vi "CAN Wrapper.vi"(5 "Signal Write":dbl, 7 "States":T1=enum."Close", 8 "error in":errorcluster, 9 "Setting":T2={"Termination"=1, "Baud Rate"=125000, "Interface"="CAN1", "XNET Database"="can_messages_818", "ECU"="GIP\ncan_messages_818"} {"Termination" items=["Off", "On"]}, 10 "Tx Signal In":string="GIP_TestMode.GIP_TestModeFlag", 11 "Rx Signal In":string) -> (0 "error out":errorcluster, 3 "Signal out":dbl=nan)   [LabVIEW 2021, in "CAN wrapper.lvlib"]
uses:
  CAN wrapper.lvlib
  Private Controls/Setting.ctl
  Private Controls/CAN States.ctl
  Private Controls/Local Variables.ctl
  <vilib>/JDP Science/JSONtext/Next JSON Value.vi
  <vilib>/JDP Science/JSONtext/String Subset.vi
  <vilib>/JDP Science/JSONtext/Parsing/Advance past next JSON Value (inlined COPY).vi
  <vilib>/JDP Science/JSONtext/Parsing/Advance past whitespace.vi
  <vilib>/JDP Science/JSONtext/Parsing/Advance past String.vi
  <vilib>/JDP Science/JSONtext/Parsing/Advance past Number.vi
  <vilib>/JDP Science/JSONtext/Parsing/Advance past Line Ending.vi
  <vilib>/xnet/xnet.llb/XNET Create Session (Signal Input Single-point).vi
  <vilib>/xnet/xnet.llb/XNET Read (Signal Single-point).vi
  <vilib>/xnet/xnet.llb/XNET Create Session (Signal Output Single-point).vi
  <vilib>/JDP Science/JSONtext/Parsing/Parse Full Path or Item Name.vi
  <vilib>/JDP Science/JSONtext/Parsing/Advance past Array.vi
  <vilib>/JDP Science/JSONtext/Parsing/Advance past Object.vi
  <vilib>/JDP Science/JSONtext/support/Error Cluster From Code.vi
  <vilib>/JDP Science/JSONtext/Offset/Find Item Locations by Path.vi
  <vilib>/xnet/xnet.llb/XNET Write (Signal Single-point).vi
  <resource>/objmgr/xnet.rc
  <vilib>/JDP Science/JSONtext/JSONtext.lvlib
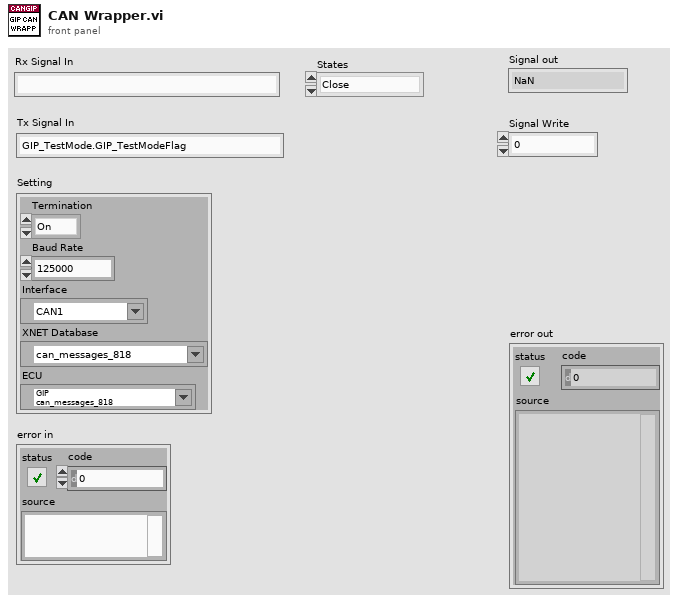
[diagram p1: front panel]
types:
  T1 = typedef "CAN wrapper.lvlib/CAN States.ctl" = enum16{"Init", "Rx Sess", "Tx Sess", "Read Signals", "Write Signals", "Close"}
  T2 = typedef "CAN wrapper.lvlib/Setting.ctl" = cluster{"Termination":u32, "Baud Rate":u64, "Interface":refnum<k21>, "XNET Database":refnum<k21>, "ECU":refnum<k21>}
  T3 = typedef "CAN wrapper.lvlib/Local Variables.ctl" = cluster{"Rx session":refnum<k21>, "Tx session":refnum<k21>, "Tx Data":dbl[], "JSON":string, "Tx Sigs":refnum<k21>[], "Rx Sigs":refnum<k21>[]}
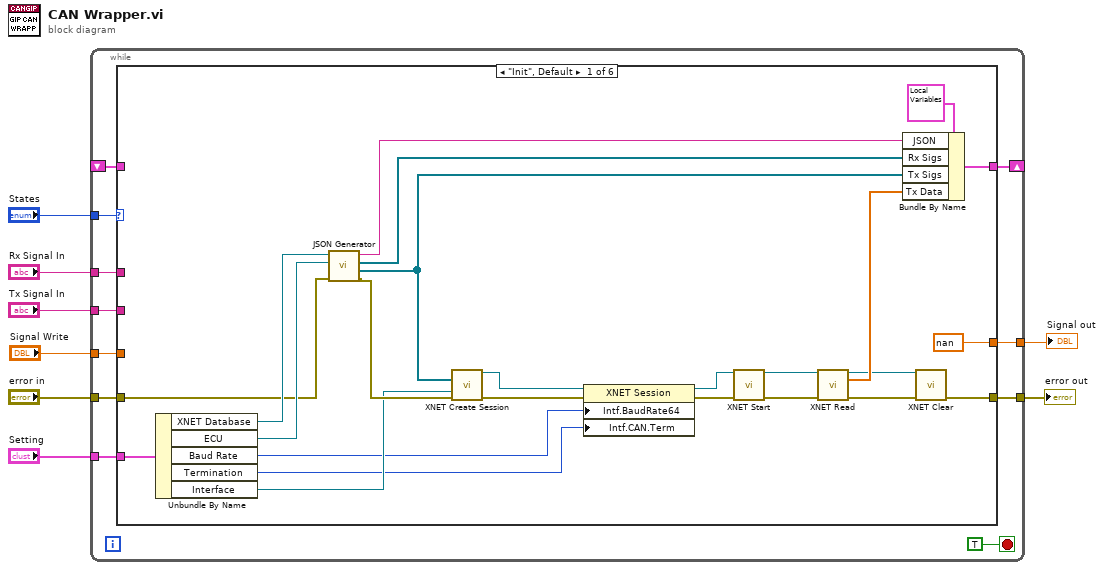
[diagram p0: block diagram]
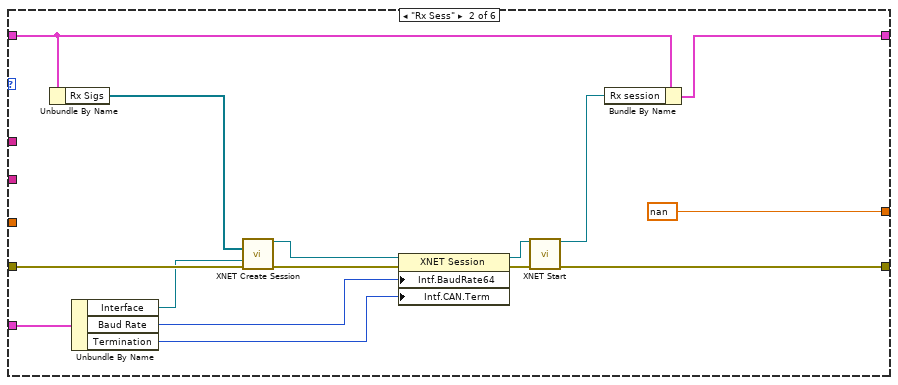
[diagram p2: hidden frame]
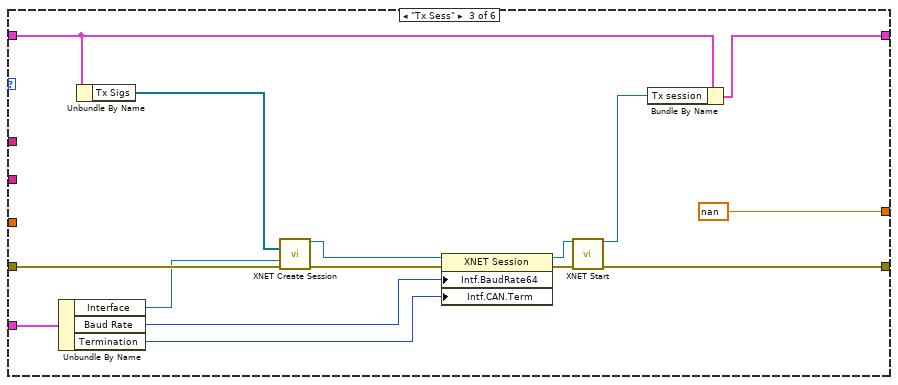
[diagram p3: hidden frame]
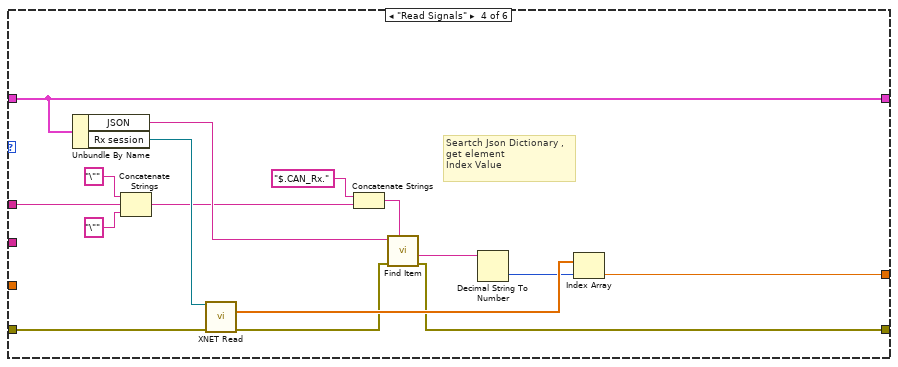
[diagram p4: hidden frame]
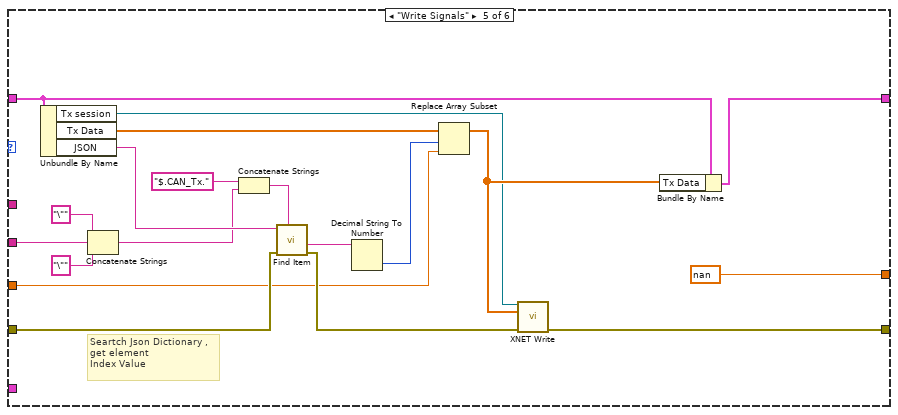
[diagram p5: hidden frame]
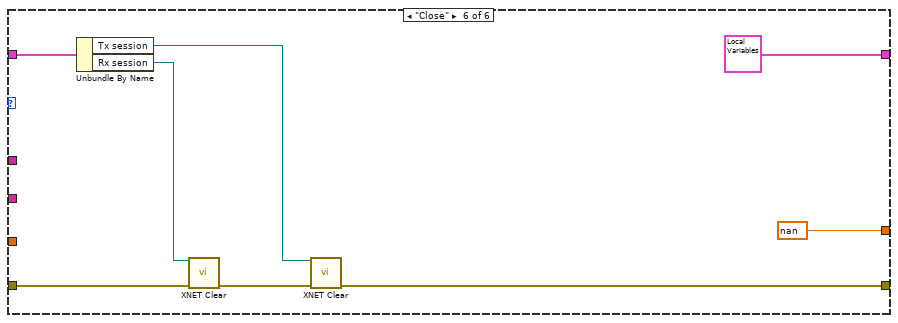
[diagram p6: hidden frame]
diagram:
  n1 = while {
    tunnel: "States" -> [w18]
    tunnel: "error in" -> [w17]
    tunnel: [w16] -> w7
    shift-right: [w15] -> _
    shift-left: _ -> [w14]
    tunnel: "Setting" -> [w13]
    tunnel: "Rx Signal In" -> [w12]
    tunnel: [w11] -> w3
    tunnel: "Signal Write" -> [w10]
    tunnel: "Tx Signal In" -> [w9]
    stop <- TRUE stop-if-true
    n2 = case shown="\"Init\", Default" w18 {
      tunnel: w17 -> [w31 w50 w68 w89 w102 w116]
      tunnel: [w21 w48 w64 w80 w90 w113] -> w16
      tunnel: [w30 w58 w65 w87 w96 T3 {"Rx session"="", "Tx session"="", "Tx Data"=[], "JSON"="{\n  \"CAN_Rx\":{\n    \"GIP_GetPartNumber.lChar0\":0,\n    \"GIP_GetPartNumber.lChar1\":1,\n    \"GIP_GetPartNumber.lChar2\":2,\n    \"GIP_GetPartNumber.lChar3\":3,\n    \"GIP_GetPartNumber.lChar4\":4,\n    \"GIP_GetPartNumber.lChar5\":5,\n    \"GIP_GetPartNumber.lChar6\":6,\n    \"GIP_GetPartNumber.lChar7\":7,\n    \"GIP_GetPartNumber.rChar0\":8,\n    \"GIP_GetPartNumber.rChar1\":9,\n    \"GIP_GetSerialNumber.vendorChar0\":10,\n    \"GIP_GetSerialNumber.vendorChar1\":11,\n    \"GIP_GetSerialNumber.vendorChar2\":12,\n    \"GIP_GetSerialNumber.weekAndSerial\":13,\n    \"GIP_Grid_ActiveEnergyExported.GIP_Grid_ActiveEnergyExported_L1\":14,\n    \"GIP_Grid_ActiveEnergyExported.GIP_Grid_ActiveEnergyExported_L2\":15,\n    \"GIP_Grid_ActiveEnergyImported.GIP_Grid_ActiveEnergyImported_L1\":16,\n    \"GIP_Grid_ActiveEnergyImported.GIP_Grid_ActiveEnergyImported_L2\":17,\n    \"GIP_Grid_Power.GIP_Grid_ActivePower_L1\":18,\n    \"GIP_Grid_Power.GIP_Grid_ActivePower_L2\":19,\n    \"GIP_Grid_Power.GIP_Grid_ReactivePower_L1\":20,\n    \"GIP_Grid_Power.GIP_Grid_ReactivePower_L2\":21,\n    \"GIP_Grid_TotalActiveEnergy.GIP_Grid_TotalActiveEnergyExported\":22,\n    \"GIP_Grid_TotalActiveEnergy.GIP_Grid_TotalActiveEnergyImported\":23,\n    \"GIP_Load_ActiveEnergyExported.GIP_Load_ActiveEnergyExported_L1\":24,\n    \"GIP_Load_ActiveEnergyExported.GIP_Load_ActiveEnergyExported_L2\":25,\n    \"GIP_Load_ActiveEnergyImported.GIP_Load_ActiveEnergyImported_L1\":26,\n    \"GIP_Load_ActiveEnergyImported.GIP_Load_ActiveEnergyImported_L2\":27,\n    \"GIP_Load_Power.GIP_Load_ActivePower_L1\":28,\n    \"GIP_Load_Power.GIP_Load_ActivePower_L2\":29,\n    \"GIP_Load_Power.GIP_Load_ReactivePower_L1\":30,\n    \"GIP_Load_Power.GIP_Load_ReactivePower_L2\":31,\n    \"GIP_Load_TotalActiveEnergy.GIP_Load_TotalActiveEnergyExported\":32,\n    \"GIP_Load_TotalActiveEnergy.GIP_Load_TotalActiveEnergyImported\":33,\n    \"GIP_Status.GIP_Relay_State\":34,\n    \"GIP_Status.GIP_State\":35\n  },\n  \"CAN_Tx\":{\n    \"GIP_ManufacturingControl.ESP32Comms\":0,\n    \"GIP_ManufacturingControl.FaultLED\":1,\n    \"GIP_ManufacturingControl.Relay\":2,\n    \"GIP_ManufacturingControl.ST8500Comms\":3,\n    \"GIP_ManufacturingControl.StatusLED\":4,\n    \"GIP_SetPartNumber.lChar0\":5,\n    \"GIP_SetPartNumber.lChar1\":6,\n    \"GIP_SetPartNumber.lChar2\":7,\n    \"GIP_SetPartNumber.lChar3\":8,\n    \"GIP_SetPartNumber.lChar4\":9,\n    \"GIP_SetPartNumber.lChar5\":10,\n    \"GIP_SetPartNumber.lChar6\":11,\n    \"GIP_SetPartNumber.lChar7\":12,\n    \"GIP_SetPartNumber.rChar0\":13,\n    \"GIP_SetPartNumber.rChar1\":14,\n    \"GIP_SetSerialNumber.vendorChar0\":15,\n    \"GIP_SetSerialNumber.vendorChar1\":16,\n    \"GIP_SetSerialNumber.vendorChar2\":17,\n    \"GIP_SetSerialNumber.weekAndSerial\":18,\n    \"GIP_SetTestedFlag.GIP_TestedFlag\":19,\n    \"GIP_TestMode.GIP_TestModeFlag\":20\n  }\n}", "Tx Sigs"=[], "Rx Sigs"=[]}] -> w15
      tunnel: w14 -> [_ w49 w67 w87 w99 w115]
      tunnel: w13 -> [w32 w47 w62 _ _ _]
      tunnel: w12 -> [_ _ _ w75 _ _]
      tunnel: [nan nan nan w85 nan nan] -> w11
      tunnel: w10 -> [_ _ _ _ w100 _]
      tunnel: w9 -> [_ _ _ _ w94 _]
      frame "Init", Default {
        n3 = Unbundle By Name(w32) -> ("XNET Database"=w42:refnum<k21>, "ECU"=w41:refnum<k21>, "Baud Rate"=w34:u64, "Termination"=w33:u32, "Interface"=w39:refnum<k21>)
        n4 = call "JSON Generator.vi"("error in (no error)"=w31, "ECU"=w41, "XNET Database"=w42) -> ("error out"=w40:errorcluster, "Tx Sigs"=w23:refnum<k21>[], "Rx Sigs"=w24:refnum<k21>[], "JSON"=w26:string)  [unwired: 5 in]
        n5 = call-poly <vilib>:"XNET Create Session.vi"("signal list"=w23, "interface"=w39, "error in (no error)"=w40) -> ("session out"=w37:refnum<k21>, "error out"=w35:errorcluster)  [unwired: 11 out]
        n6 = property class="XNET Session"(reference=w37, error in=w35, "Intf.BaudRate64"=w34, "Intf.CAN.Term"=w33) -> (reference out=w36:refnum<k21>, error out=w38:errorcluster)
        n7 = call <vilib>:"XNET Start.vi"("session in"=w36, "error in (no error)"=w38) -> ("session out"=w28:refnum<k21>, "error out"=w29:errorcluster)  [unwired: 12 in]
        n8 = call-poly <vilib>:"XNET Read.vi"("session in"=w28, "error in (no error)"=w29) -> ("session out"=w20:refnum<k21>, "data"=w27:dbl[], "error out"=w22:errorcluster)  [unwired: 11 out]
        n9 = Bundle By Name(cluster=T3 {"Rx session"="", "Tx session"="", "Tx Data"=[], "JSON"="{\n  \"CAN_Rx\":{\n    \"GIP_GetPartNumber.lChar0\":0,\n    \"GIP_GetPartNumber.lChar1\":1,\n    \"GIP_GetPartNumber.lChar2\":2,\n    \"GIP_GetPartNumber.lChar3\":3,\n    \"GIP_GetPartNumber.lChar4\":4,\n    \"GIP_GetPartNumber.lChar5\":5,\n    \"GIP_GetPartNumber.lChar6\":6,\n    \"GIP_GetPartNumber.lChar7\":7,\n    \"GIP_GetPartNumber.rChar0\":8,\n    \"GIP_GetPartNumber.rChar1\":9,\n    \"GIP_GetSerialNumber.vendorChar0\":10,\n    \"GIP_GetSerialNumber.vendorChar1\":11,\n    \"GIP_GetSerialNumber.vendorChar2\":12,\n    \"GIP_GetSerialNumber.weekAndSerial\":13,\n    \"GIP_Grid_ActiveEnergyExported.GIP_Grid_ActiveEnergyExported_L1\":14,\n    \"GIP_Grid_ActiveEnergyExported.GIP_Grid_ActiveEnergyExported_L2\":15,\n    \"GIP_Grid_ActiveEnergyImported.GIP_Grid_ActiveEnergyImported_L1\":16,\n    \"GIP_Grid_ActiveEnergyImported.GIP_Grid_ActiveEnergyImported_L2\":17,\n    \"GIP_Grid_Power.GIP_Grid_ActivePower_L1\":18,\n    \"GIP_Grid_Power.GIP_Grid_ActivePower_L2\":19,\n    \"GIP_Grid_Power.GIP_Grid_ReactivePower_L1\":20,\n    \"GIP_Grid_Power.GIP_Grid_ReactivePower_L2\":21,\n    \"GIP_Grid_TotalActiveEnergy.GIP_Grid_TotalActiveEnergyExported\":22,\n    \"GIP_Grid_TotalActiveEnergy.GIP_Grid_TotalActiveEnergyImported\":23,\n    \"GIP_Load_ActiveEnergyExported.GIP_Load_ActiveEnergyExported_L1\":24,\n    \"GIP_Load_ActiveEnergyExported.GIP_Load_ActiveEnergyExported_L2\":25,\n    \"GIP_Load_ActiveEnergyImported.GIP_Load_ActiveEnergyImported_L1\":26,\n    \"GIP_Load_ActiveEnergyImported.GIP_Load_ActiveEnergyImported_L2\":27,\n    \"GIP_Load_Power.GIP_Load_ActivePower_L1\":28,\n    \"GIP_Load_Power.GIP_Load_ActivePower_L2\":29,\n    \"GIP_Load_Power.GIP_Load_ReactivePower_L1\":30,\n    \"GIP_Load_Power.GIP_Load_ReactivePower_L2\":31,\n    \"GIP_Load_TotalActiveEnergy.GIP_Load_TotalActiveEnergyExported\":32,\n    \"GIP_Load_TotalActiveEnergy.GIP_Load_TotalActiveEnergyImported\":33,\n    \"GIP_Status.GIP_Relay_State\":34,\n    \"GIP_Status.GIP_State\":35\n  },\n  \"CAN_Tx\":{\n    \"GIP_ManufacturingControl.ESP32Comms\":0,\n    \"GIP_ManufacturingControl.FaultLED\":1,\n    \"GIP_ManufacturingControl.Relay\":2,\n    \"GIP_ManufacturingControl.ST8500Comms\":3,\n    \"GIP_ManufacturingControl.StatusLED\":4,\n    \"GIP_SetPartNumber.lChar0\":5,\n    \"GIP_SetPartNumber.lChar1\":6,\n    \"GIP_SetPartNumber.lChar2\":7,\n    \"GIP_SetPartNumber.lChar3\":8,\n    \"GIP_SetPartNumber.lChar4\":9,\n    \"GIP_SetPartNumber.lChar5\":10,\n    \"GIP_SetPartNumber.lChar6\":11,\n    \"GIP_SetPartNumber.lChar7\":12,\n    \"GIP_SetPartNumber.rChar0\":13,\n    \"GIP_SetPartNumber.rChar1\":14,\n    \"GIP_SetSerialNumber.vendorChar0\":15,\n    \"GIP_SetSerialNumber.vendorChar1\":16,\n    \"GIP_SetSerialNumber.vendorChar2\":17,\n    \"GIP_SetSerialNumber.weekAndSerial\":18,\n    \"GIP_SetTestedFlag.GIP_TestedFlag\":19,\n    \"GIP_TestMode.GIP_TestModeFlag\":20\n  }\n}", "Tx Sigs"=[], "Rx Sigs"=[]}, "JSON"=w26, "Rx Sigs"=w24, "Tx Sigs"=w23, "Tx Data"=w27) -> (w30:T3)
        n10 = call <vilib>:"XNET Clear.vi"("session in"=w20, "error in (no error)"=w22) -> ("error out"=w21:errorcluster)  [unwired: 13 in]
      }
      frame "Rx Sess" {
        n11 = Unbundle By Name(w49) -> ("Rx Sigs"=w51:refnum<k21>[])
        n12 = Unbundle By Name(w47) -> ("Interface"=w44:refnum<k21>, "Baud Rate"=w46:u64, "Termination"=w45:u32)
        n13 = call-poly <vilib>:"XNET Create Session.vi"("signal list"=w51, "interface"=w44, "error in (no error)"=w50) -> ("session out"=w55:refnum<k21>, "error out"=w53:errorcluster)  [unwired: 11 out]
        n14 = property class="XNET Session"(reference=w55, error in=w53, "Intf.BaudRate64"=w46, "Intf.CAN.Term"=w45) -> (reference out=w54:refnum<k21>, error out=w56:errorcluster)
        n15 = call <vilib>:"XNET Start.vi"("session in"=w54, "error in (no error)"=w56) -> ("session out"=w52:refnum<k21>, "error out"=w48:errorcluster)  [unwired: 12 in]
        n16 = Bundle By Name(cluster=w49, "Rx session"=w52) -> (w58:T3)
      }
      frame "Tx Sess" {
        n17 = Unbundle By Name(w62) -> ("Interface"=w59:refnum<k21>, "Baud Rate"=w61:u64, "Termination"=w60:u32)
        n18 = Unbundle By Name(w67) -> ("Tx Sigs"=w69:refnum<k21>[])
        n19 = call-poly <vilib>:"XNET Create Session.vi"("signal list"=w69, "interface"=w59, "error in (no error)"=w68) -> ("session out"=w70:refnum<k21>, "error out"=w71:errorcluster)  [unwired: 11 out]
        n20 = property class="XNET Session"(reference=w70, error in=w71, "Intf.BaudRate64"=w61, "Intf.CAN.Term"=w60) -> (reference out=w73:refnum<k21>, error out=w72:errorcluster)
        n21 = call <vilib>:"XNET Start.vi"("session in"=w73, "error in (no error)"=w72) -> ("session out"=w66:refnum<k21>, "error out"=w64:errorcluster)  [unwired: 12 in]
        n22 = Bundle By Name(cluster=w67, "Tx session"=w66) -> (w65:T3)
      }
      frame "Read Signals" {
        # "Seartch Json Dictionary ,\nget element\nIndex Value"
        n23 = Unbundle By Name(w87) -> ("JSON"=w82:string, "Rx session"=w88:refnum<k21>)
        n24 = Concatenate Strings("\"" ("string"), w75, "\"" ("string")) -> (w74:string)
        n25 = call-poly <vilib>:"XNET Read.vi"("session in"=w88, "error in (no error)"=w89) -> ("data"=w86:dbl[], "error out"=w81:errorcluster)  [unwired: 12 out]
        n26 = Concatenate Strings("$.CAN_Rx." ("$Path or Item Name"), w74) -> (w83:string)
        n27 = call <vilib>:"Find Item.vi"("$Path or Item Name"=w83, "error in (no error)"=w81, "JSON"=w82) -> ("error out"=w80:errorcluster, "<JSON>"=w78:string)  [unwired: 5 in, 2 out]
        n28 = Decimal String To Number(string=w78) -> (number=w79:i32)  [unwired: 2 in, 1 out]
        n29 = Index Array(array=w86, index=w79) -> (element=w85:dbl)
      }
      frame "Write Signals" {
        # "Seartch Json Dictionary ,\nget element\nIndex Value"
        n30 = Unbundle By Name(w99) -> ("Tx session"=w95:refnum<k21>, "Tx Data"=w98:dbl[], "JSON"=w104:string)
        n31 = Concatenate Strings("\"" ("string"), w94, "\"" ("string")) -> (w92:string)
        n32 = Concatenate Strings("$.CAN_Tx." ("$Path or Item Name"), w92) -> (w105:string)
        n33 = call <vilib>:"Find Item.vi"("$Path or Item Name"=w105, "error in (no error)"=w102, "JSON"=w104) -> ("error out"=w101:errorcluster, "<JSON>"=w107:string)  [unwired: 5 in, 2 out]
        n34 = Decimal String To Number(string=w107) -> (number=w103:i32)  [unwired: 2 in, 1 out]
        n35 = Replace Array Subset(array=w98, new element=w100, index=w103) -> (w97:dbl[])
        n36 = call-poly <vilib>:"XNET Write.vi"("session in"=w95, "data"=w97, "error in (no error)"=w101) -> ("error out"=w90:errorcluster)  [unwired: 12 out]
        n37 = Bundle By Name(cluster=w99, "Tx Data"=w97) -> (w96:T3)
      }
      frame "Close" {
        n38 = Unbundle By Name(w115) -> ("Tx session"=w111:refnum<k21>, "Rx session"=w112:refnum<k21>)
        n39 = call <vilib>:"XNET Clear.vi"("session in"=w112, "error in (no error)"=w116) -> ("error out"=w114:errorcluster)  [unwired: 13 in]
        n40 = call <vilib>:"XNET Clear.vi"("session in"=w111, "error in (no error)"=w114) -> ("error out"=w113:errorcluster)  [unwired: 13 in]
      }
    }
  }
  "error out" <- w7
  "Signal out" <- w3
